vi "createLabelErrors.vi"(1 "N modules":i32) -> (0 "labels (out)":string[](array[string]))   [LabVIEW 2021]
panel:
  in  "labels":string[](array[string])=["Time UTC", "I_src", "V_src", "BMS_Vbat", "BMS_Ibat", "BMS_SoC", "BMS_SoH"]
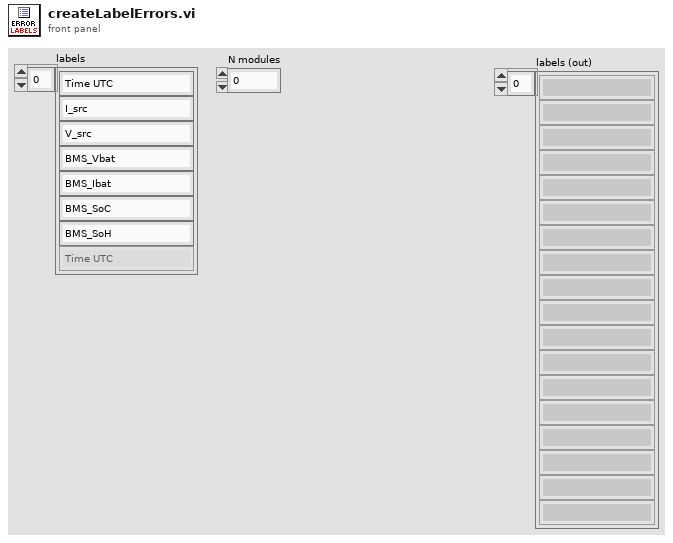
[diagram p1: front panel]
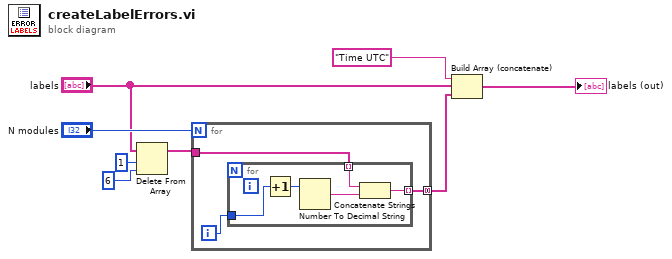
[diagram p0: block diagram]
diagram:
  n1 = Delete From Array(array="labels", length=1, index=6) -> (array with subset deleted=w3:string[])  [unwired: 1 out]
  n2 = for {
    N: "N modules" -> [_]
    tunnel: w3 -> [w11]
    tunnel: [w10] -> w7 mode=concatenating
    i -> [w9]
    n3 = for {
      tunnel: [w16] -> w10 mode=indexing
      tunnel: w11 -> [w13] mode=indexing
      tunnel: w9 -> [w12]
      n4 = Increment(x=w12) -> (x+1=w15:i32)
      n5 = Number To Decimal String(number=w15) -> (decimal integer string=w14:string)  [unwired: 1 in]
      n6 = Concatenate Strings(w13, w14) -> (w16:string)
    }
  }
  n7 = Build Array (concatenate)("Time UTC", "labels", w7) -> (→"labels (out)":string[])
